vi "Example_analog_out_control.vi"() -> ()   [LabVIEW 2022 SP3]
uses:
  usbtmc_scpi_labtool.lvlib
panel:
  in  "ID Query (True)":bool=TRUE
  in  "ID query string":string="PICO-PI,LABTOOL"
  in  "stop":bool
  in  "set duty cycle":i16(slide) min=0 max=4095 step=1 scale=0.0..4095.0
  out "read duty cycle":i16(slide) scale=0.0..4095.0
  in  "VISA resource name in":refnum<visa-resource-name>
  in  "Pin":u8 max=7 step=1
  # "In this example, you control the \nduty cycle of the selected pin with\nthe slider at left. The value is also read \nback  and displayed on the bar above."
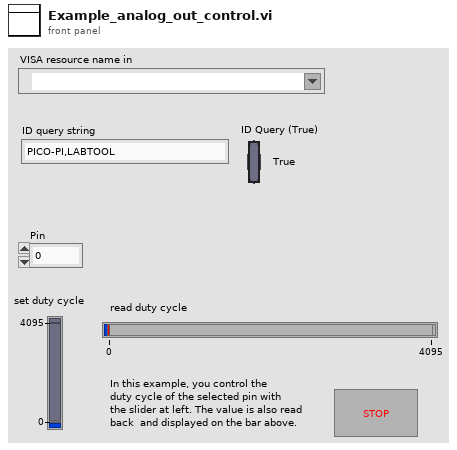
[diagram p1: front panel]
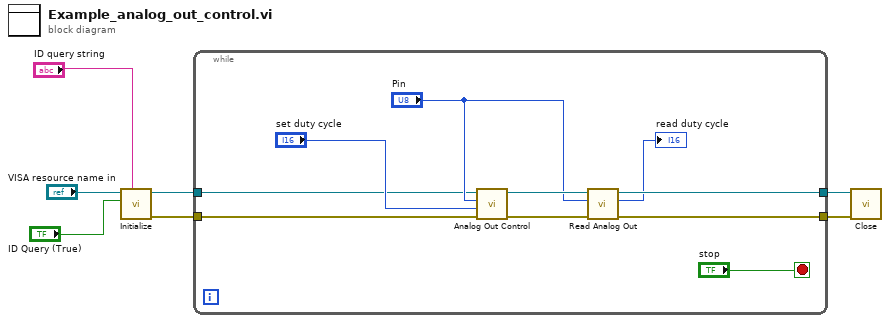
[diagram p0: block diagram]
diagram:
  n1 = call "Initialize.vi"("ID query string"="ID query string", "ID Query (True)"="ID Query (True)", "VISA resource name in"="VISA resource name in") -> ("error out"=w5:errorcluster, "VISA resource name out"=w7:refnum<visa-resource-name>)  [unwired: 7 in]
  n2 = while {
    tunnel: w7 -> [w10]
    tunnel: [w17] -> w6
    tunnel: w5 -> [w9]
    tunnel: [w16] -> w4
    stop <- "stop" stop-if-true
    n3 = call "Analog Out Control.vi"("VISA resource name"=w10, "Pin"="Pin", "duty cycle"="set duty cycle", "error in (no error)"=w9) -> ("VISA resource name out"=w15:refnum<visa-resource-name>, "error out"=w14:errorcluster)  [unwired: 5 in]
    n4 = call "Read Analog Out.vi"("error in (no error)"=w14, "Pin"="Pin", "VISA resource name"=w15) -> ("error out"=w16:errorcluster, "duty cycle"=→"read duty cycle":i16, "VISA resource name out"=w17:refnum<visa-resource-name>)  [unwired: 6 in]
  }
  n5 = call "Close.vi"("error in (no error)"=w4, "VISA resource name"=w6) -> ()  [unwired: 10 in]
